vi "Database.Tools.RecognizeParameter(NaN).vi"(9 "Type Enum":T1, 11 "Variant data in":variant) -> (3 "Variant data out":variant)   [LabVIEW 2016]
uses:
  <vilib>/Utility/VariantDataType/Type.ctl
  <vilib>/Utility/VariantDataType/VariantType.lvlib
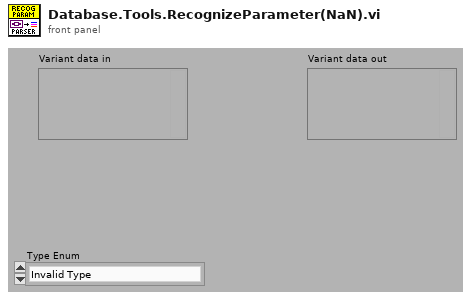
[diagram p1: front panel]
types:
  T1 = typedef "VariantType.lvlib/Type.ctl" = enum8{"Invalid Type", "Void", "I8", "I16", "I32", "I64", "U8", "U16", "U32", "U64", "Single Float", "Double Float", "Extended Float", "Single Complex", "Double Complex", "Extended Complex", "Enum U8", "Enum U16", "Enum U32", "Enum U64", "Single Float With Unit", "Double Float With Unit", "Extended Float With Unit", "Single Complex with Unit", "Double Complex with Unit", "Extended Complex with Unit", "Boolean", "String", "Path", "Picture", "Tag", "Array", "Cluster", "Variant", "LV Variant", "Waveform", "Timestamp", "Digital Waveform", "Digital Data", "ExpressData", "Refnum", "External Data", "VI", "Poly VI", "LabVIEW Class Instance", "Fixed Point"}
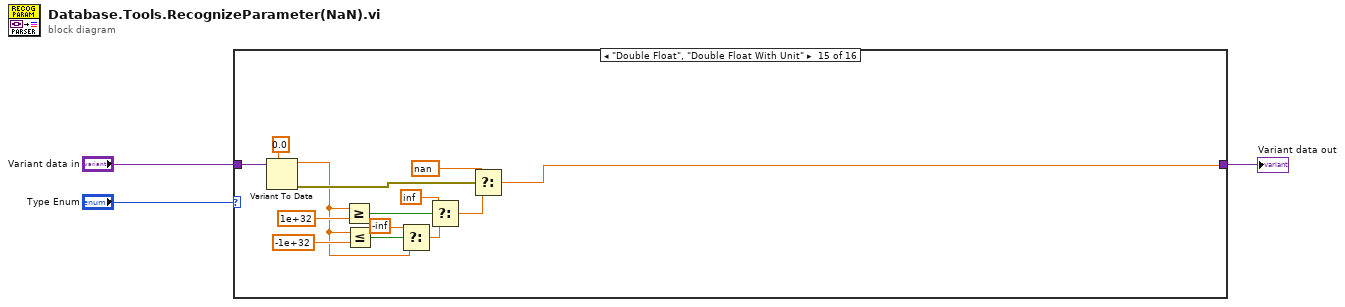
[diagram p0: block diagram]
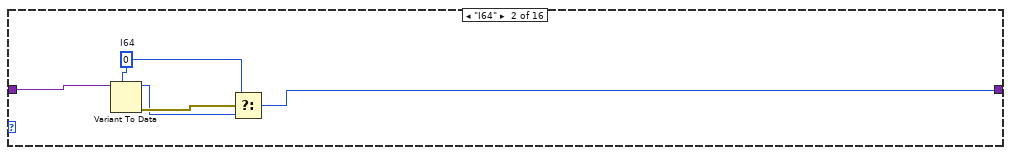
[diagram p3: hidden frame]
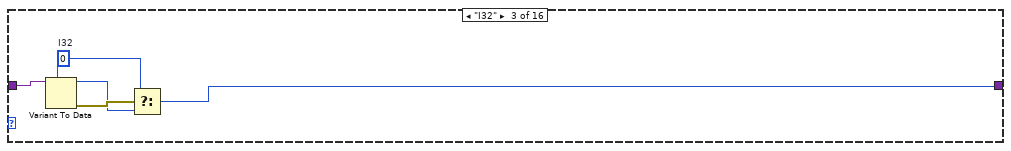
[diagram p4: hidden frame]
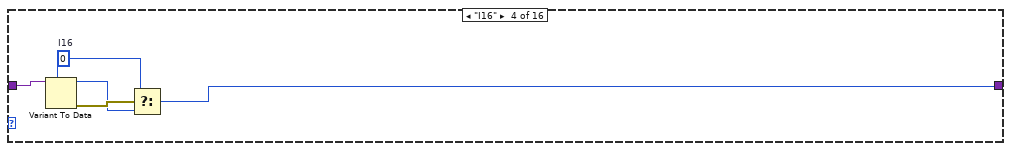
[diagram p5: hidden frame]
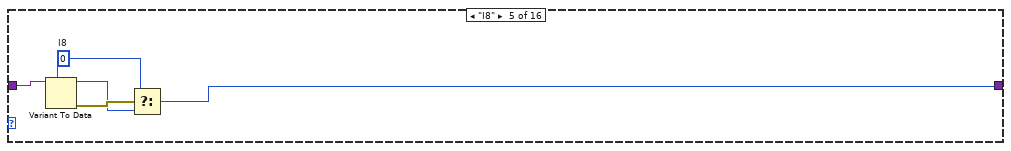
[diagram p6: hidden frame]
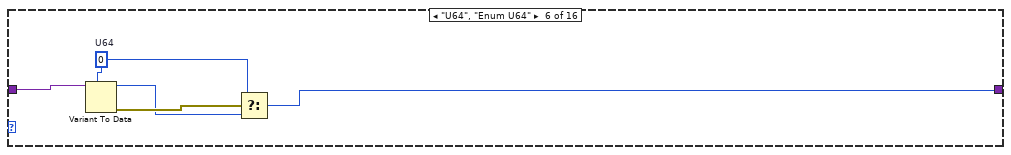
[diagram p7: hidden frame]
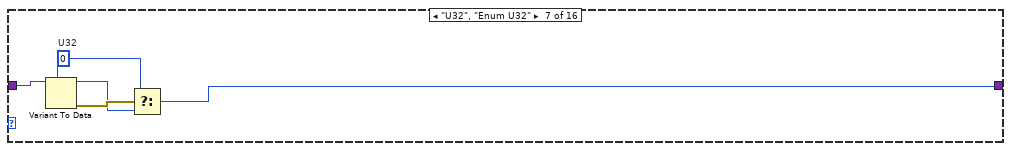
[diagram p8: hidden frame]
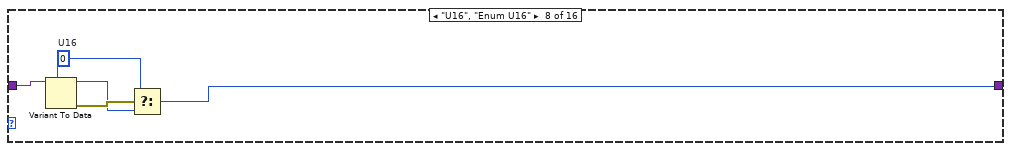
[diagram p9: hidden frame]
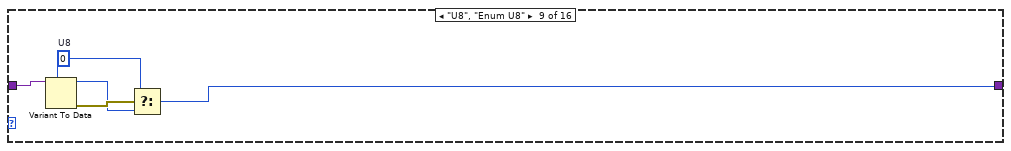
[diagram p10: hidden frame]
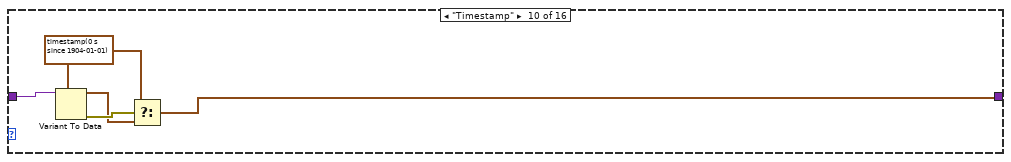
[diagram p11: hidden frame]
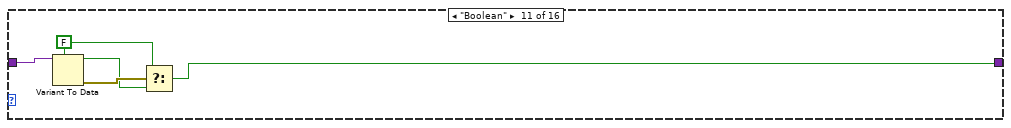
[diagram p12: hidden frame]
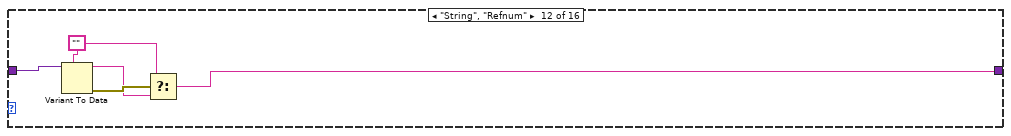
[diagram p13: hidden frame]
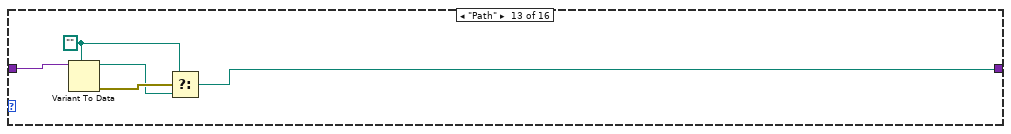
[diagram p14: hidden frame]
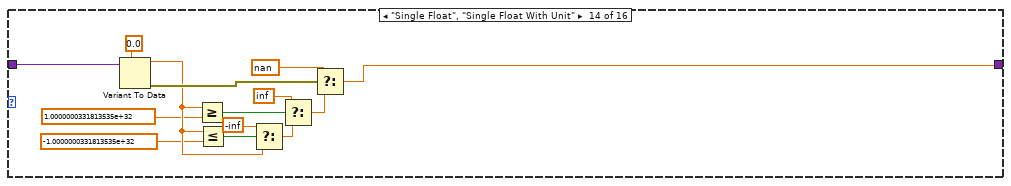
[diagram p15: hidden frame]
diagram:
  n1 = case shown="\"Double Float\", \"Double Float With Unit\"" "Type Enum" {
    tunnel: "Variant data in" -> [w4 w9 w12 w17 w22 w29 w32 w37 w42 w49 w54 w59 w64 w68 w91 w93]
    tunnel: [w4 w5 w10 w15 w20 w25 w30 w35 w40 w45 w50 w55 w60 w65 w79 w93] -> w1
    frame "Invalid Type", "Void", "Tag" {
    }
    frame "I64" {
      w7 = i64 0  # I64
      n2 = Variant To Data(type=w7, Variant=w9) -> (data=w6:i64, error out=w8:errorcluster)  [unwired: 1 in]
      n3 = Select(t=w7, s=w8, f=w6) -> (s? t:f=w5:i64)
    }
    frame "I32" {
      w11 = 0  # I32
      n4 = Variant To Data(type=w11, Variant=w12) -> (data=w13:i32, error out=w14:errorcluster)  [unwired: 1 in]
      n5 = Select(t=w11, s=w14, f=w13) -> (s? t:f=w10:i32)
    }
    frame "I16" {
      w16 = i16 0  # I16
      n6 = Variant To Data(type=w16, Variant=w17) -> (data=w18:i16, error out=w19:errorcluster)  [unwired: 1 in]
      n7 = Select(t=w16, s=w19, f=w18) -> (s? t:f=w15:i16)
    }
    frame "I8" {
      w21 = i8 0  # I8
      n8 = Variant To Data(type=w21, Variant=w22) -> (data=w23:i8, error out=w24:errorcluster)  [unwired: 1 in]
      n9 = Select(t=w21, s=w24, f=w23) -> (s? t:f=w20:i8)
    }
    frame "U64", "Enum U64" {
      w26 = u64 0  # U64
      n10 = Variant To Data(type=w26, Variant=w29) -> (data=w27:u64, error out=w28:errorcluster)  [unwired: 1 in]
      n11 = Select(t=w26, s=w28, f=w27) -> (s? t:f=w25:u64)
    }
    frame "U32", "Enum U32" {
      w31 = u32 0  # U32
      n12 = Variant To Data(type=w31, Variant=w32) -> (data=w33:u32, error out=w34:errorcluster)  [unwired: 1 in]
      n13 = Select(t=w31, s=w34, f=w33) -> (s? t:f=w30:u32)
    }
    frame "U16", "Enum U16" {
      w36 = u16 0  # U16
      n14 = Variant To Data(type=w36, Variant=w37) -> (data=w38:u16, error out=w39:errorcluster)  [unwired: 1 in]
      n15 = Select(t=w36, s=w39, f=w38) -> (s? t:f=w35:u16)
    }
    frame "U8", "Enum U8" {
      w41 = u8 0  # U8
      n16 = Variant To Data(type=w41, Variant=w42) -> (data=w43:u8, error out=w44:errorcluster)  [unwired: 1 in]
      n17 = Select(t=w41, s=w44, f=w43) -> (s? t:f=w40:u8)
    }
    frame "Timestamp" {
      w46 = timestamp(0 s since 1904-01-01)
      n18 = Variant To Data(type=w46, Variant=w49) -> (data=w47:timestamp, error out=w48:errorcluster)  [unwired: 1 in]
      n19 = Select(t=w46, s=w48, f=w47) -> (s? t:f=w45:timestamp)
    }
    frame "Boolean" {
      w51 = FALSE ("Boolean")
      n20 = Variant To Data(type=w51, Variant=w54) -> (data=w52:bool, error out=w53:errorcluster)  [unwired: 1 in]
      n21 = Select(t=w51, s=w53, f=w52) -> (s? t:f=w50:bool)
    }
    frame "String", "Refnum" {
      w56 = ""
      n22 = Variant To Data(type=w56, Variant=w59) -> (data=w57:string, error out=w58:errorcluster)  [unwired: 1 in]
      n23 = Select(t=w56, s=w58, f=w57) -> (s? t:f=w55:string)
    }
    frame "Path" {
      w61 = path ""
      n24 = Variant To Data(type=w61, Variant=w64) -> (data=w62:path, error out=w63:errorcluster)  [unwired: 1 in]
      n25 = Select(t=w61, s=w63, f=w62) -> (s? t:f=w60:path)
    }
    frame "Single Float", "Single Float With Unit" {
      n26 = Variant To Data(type=sgl 0.0, Variant=w68) -> (data=w71:sgl, error out=w77:errorcluster)  [unwired: 1 in]
      n27 = Greater Or Equal?(x=w71, y=sgl 1e+32) -> (x >= y?=w76:bool)
      n28 = Less Or Equal?(x=w71, y=sgl -1e+32) -> (x <= y?=w74:bool)
      n29 = Select(t=sgl -inf, s=w74, f=w71) -> (s? t:f=w73:sgl)
      n30 = Select(t=sgl inf, s=w76, f=w73) -> (s? t:f=w70:sgl)
      n31 = Select(t=sgl nan, s=w77, f=w70) -> (s? t:f=w65:sgl)
    }
    frame "Double Float", "Double Float With Unit" {
      n32 = Variant To Data(type=0.0, Variant=w91) -> (data=w82:dbl, error out=w90:errorcluster)  [unwired: 1 in]
      n33 = Greater Or Equal?(x=w82, y=1e+32) -> (x >= y?=w88:bool)
      n34 = Less Or Equal?(x=w82, y=-1e+32) -> (x <= y?=w85:bool)
      n35 = Select(t=-inf, s=w85, f=w82) -> (s? t:f=w84:dbl)
      n36 = Select(t=inf, s=w88, f=w84) -> (s? t:f=w81:dbl)
      n37 = Select(t=nan, s=w90, f=w81) -> (s? t:f=w79:dbl)
    }
    frame "Extended Float".."Extended Complex", "Extended Float With Unit".."Extended Complex with Unit", "Picture", "Array".."Waveform", "Digital Waveform".."ExpressData", "External Data".."Fixed Point" {
    }
  }
  "Variant data out" <- w1
